vi "sub_Gmap4_GNSS-Ntrip.vi"(8 "error in":errorcluster) -> (0 "error out":errorcluster)   [LabVIEW 2019]
uses:
  Gmap/gmap_fgv-cmd.ctl
  Gmap/marker_info.ctl
  Ctrl/error_state-val.ctl
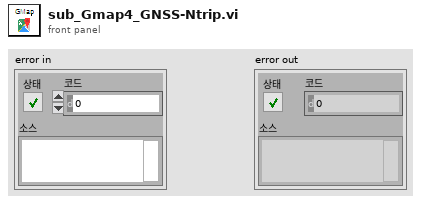
[diagram p1: front panel]
types:
  T1 = typedef "gmap_fgv-cmd.ctl" = enum16{"marker type change", "save_image", "coll of points", "zoom n center markers", "add overlay reference", "read", "zoom", "set position by keyword", "set map provider", "map provider update", "create", "add marker", "clear marker", "close"}
  T2 = typedef "marker_info.ctl" = cluster{"arrLatLngActv":dbl[], "type":i32}
  T3 = typedef "error_state-val.ctl" = enum16{"na", "error", "OK"}
  T4 = typedef "Ntrip error-leds.ctl" = cluster{"GNSS Serial":u8, "NMEA val":u8, "Send Serial":u8, "Ntrip TCP":u8, "RTCM val":u8, "GMAP":u8, "TBD1":u8, "TBD2":u8, "TBD3":u8}
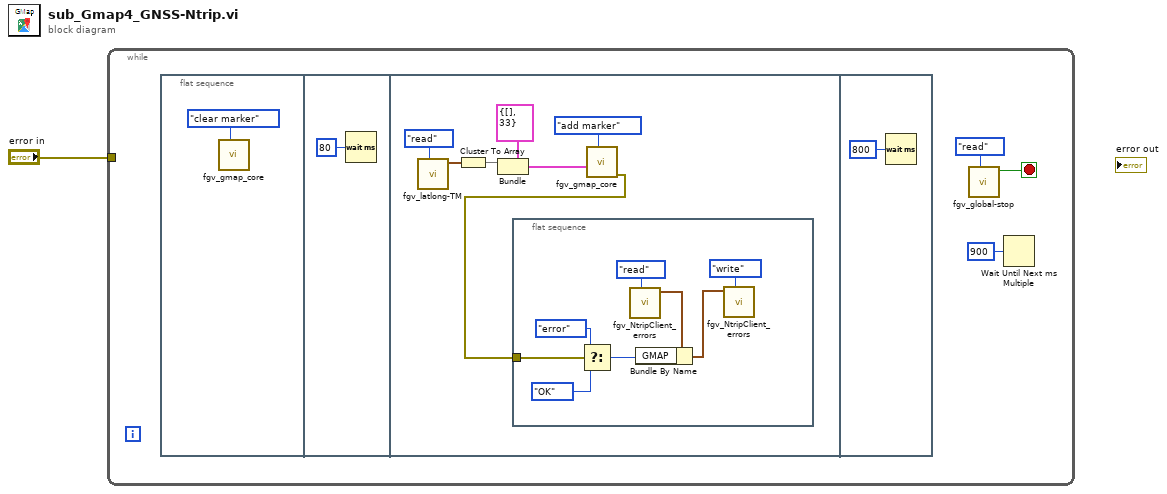
[diagram p0: block diagram]
diagram:
  n1 = while {
    tunnel: "error in" -> [_]
    stop <- w3 stop-if-true
    n2 = flat-sequence {
      frame #0 {
        n3 = call "fgv_gmap_core.vi"("cmd"=gmap_fgv-cmd."clear marker") -> ()  [unwired: 7 in, 4 out]
      }
      frame #1 {
        n4 = Wait (ms)(milliseconds to wait=u32 80 ("대기 시간 (ms)")) -> ()  [unwired: 1 out]
      }
      frame #2 {
        n5 = call "fgv_latlong-TM.vi"("cmd"=enum16{"write", "read"}."read") -> ("latlong out"=w8:cluster{"lat":dbl, "long":dbl})  [unwired: 9 in, 1 out]
        n6 = Cluster To Array(cluster=w8) -> (array=w12:dbl[])
        n7 = Bundle(cluster=T2 {"arrLatLngActv"=[], "type"=33} ("marker_info"), "arrLatLngActv"=w12) -> (w10:T2)  [unwired: 1 in]
        n8 = flat-sequence {
          tunnel: w7 -> [w17]
          frame #0 {
            n9 = Select(t=error_state-val."error", s=w17, f=error_state-val."OK") -> (s? t:f=w14:T3)
            n10 = call "fgv_NtripClient_errors.vi"("cmd"=enum16{"init", "read", "write"}."read") -> ("Error led out"=w19:T4)  [unwired: 9 in, 1 out]
            n11 = Bundle By Name(cluster=w19, "GMAP"=w14) -> (w18:T4)
            n12 = call "fgv_NtripClient_errors.vi"("cmd"=enum16{"init", "read", "write"}."write", "Error led"=w18) -> ()  [unwired: 8 in, 2 out]
          }
        }
        n13 = call "fgv_gmap_core.vi"("cmd"=gmap_fgv-cmd."add marker", "marker_info"=w10) -> ("error out"=w7:errorcluster)  [unwired: 6 in, 3 out]
      }
      frame #3 {
        n14 = Wait (ms)(milliseconds to wait=u32 800 ("대기 시간 (ms)")) -> ()  [unwired: 1 out]
      }
    }
    n15 = call "fgv_global-stop.vi"("cmd"=enum16{"init", "stop", "read"}."read") -> ("val_out"=w3:bool)  [unwired: 10 in]
    n16 = Wait Until Next ms Multiple(millisecond multiple=u32 900 ("ms 배수")) -> ()  [unwired: 1 out]
  }
